vi "SUB VI encriptación.vi"(8 "error in (no error)":errorcluster, 11 "Image 2":T1) -> (0 "error out":errorcluster, 2 "KEY ARRAY":bool[](array[boolean]), 3 "Image":T1(plugin-control))   [LabVIEW 2023]
uses:
  <vilib>/vision/Image Controls.llb/IMAQ Image.ctl
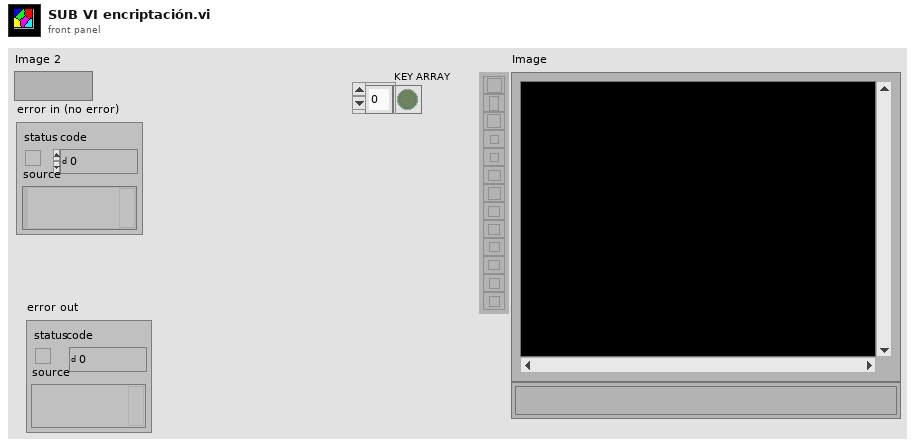
[diagram p1: front panel]
types:
  T1 = typedef "IMAQ Image.ctl" = refnum<image>
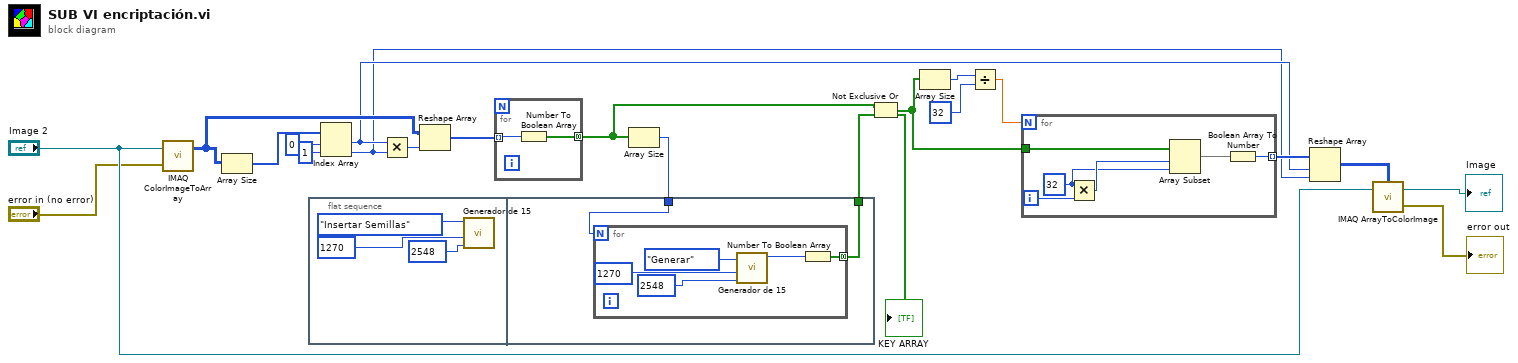
[diagram p0: block diagram]
diagram:
  n1 = call "IMAQ ColorImageToArray"("Image"="Image 2", "error in (no error)"="error in (no error)") -> ("Image Pixels (U32)"=w18:u32[][])  [unwired: 2 in, 2 out]
  n2 = Array Size(array=w18) -> (size(s)=w21:i32[])
  n3 = flat-sequence {
    tunnel: w15 -> [w26]
    tunnel: [w25] -> w14
    frame #0 {
      n4 = call "Generador de 15.vi"("Semilla 2"=u16 2548, "Semilla 1"=u16 1270, "Modo"=enum16{"Insertar Semillas", "Generar"}."Insertar Semillas") -> ()  [unwired: 8 in, 1 out]
    }
    frame #1 {
      n5 = for {
        N: w26 -> [_]
        tunnel: [w27] -> w25 mode=concatenating
        n6 = call "Generador de 15.vi"("Semilla 2"=u16 2548, "Semilla 1"=u16 1270, "Modo"=enum16{"Insertar Semillas", "Generar"}."Generar") -> ("Recorrdo"=w28:u16)  [unwired: 8 in]
        n7 = Number To Boolean Array(number=w28) -> (Boolean array=w27:bool[])
      }
    }
  }
  n8 = Index Array(array=w21, index #1=0 ("index"), index #2=1 ("index")) -> (element #1=w7:i32, element #2=w6:i32)
  n9 = Multiply(x=w7, y=w6) -> (x*y=w17:i32)
  n10 = Reshape Array(w18, w17) -> (w16:u32[])
  n11 = for {
    tunnel: w16 -> [w33] mode=indexing
    tunnel: [w32] -> w13 mode=concatenating
    n12 = Number To Boolean Array(number=w33) -> (Boolean array=w32:bool[])
  }
  n13 = Array Size(array=w13) -> (size(s)=w15:i32)
  n14 = Not Exclusive Or(1:w14, 2:w13) -> (0:w9:bool[])
  n15 = Array Size(array=w9) -> (size(s)=w12:i32)
  n16 = Divide(x=w12, y=32) -> (x/y=w10:dbl)
  n17 = for {
    N: w10 -> [_]
    tunnel: w9 -> [w39]
    tunnel: [w34] -> w8 mode=indexing
    i -> [w38]
    w36 = 32
    n18 = Multiply(x=w36, y=w38) -> (x*y=w37:i32)
    n19 = Array Subset(array=w39, index=w37, length=w36) -> (w35:bool[])
    n20 = Boolean Array To Number(Boolean array=w35) -> (number=w34:u32)
  }
  n21 = Reshape Array(w8, w7, w6) -> (w5:u32[][])
  n22 = call "IMAQ ArrayToColorImage"("Image Pixels (U32)"=w5, "Image"="Image 2") -> ("Image Out"=→"Image":T1, "error out"=→"error out":errorcluster)  [unwired: 3 in]
  "KEY ARRAY" <- w14
